vi "saveVI.vi"(8 "error in (no error)":errorcluster, 11 "PolymorphicInstance in":refnum<class "PolymorphicInstance.lvclass">) -> (0 "error out":errorcluster, 3 "PolymorphicInstance out":refnum<class "PolymorphicInstance.lvclass">)   [LabVIEW 2013, in "PolymorphicInstance.lvclass"]
uses:
  PolymorphicInstance.lvclass
  PolymorphicInstance.lvclass/PolymorphicInstance.ctl
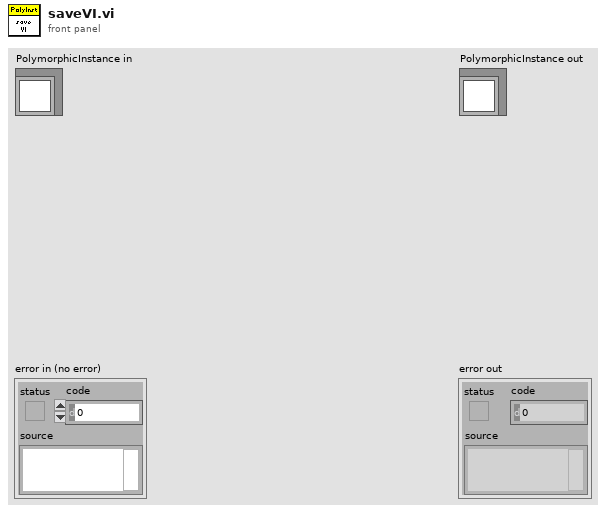
[diagram p1: front panel]
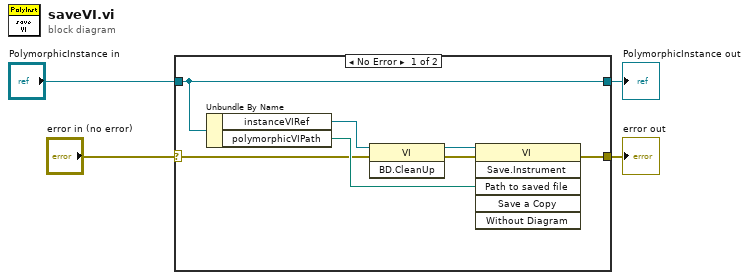
[diagram p0: block diagram]
diagram:
  n1 = case shown="No Error" "error in (no error)" {
    selector: "error in (no error)" -> [w6 w13]
    tunnel: [w5 w13] -> w3
    tunnel: [w11 w12] -> w1
    tunnel: "PolymorphicInstance in" -> [w11 w12]
    frame No Error {
      n2 = Unbundle By Name(w11) -> ("instanceVIRef"=w10:refnum<vi>, "polymorphicVIPath"=w8:path)
      n3 = invoke class="VI" method="BD.CleanUp"(reference=w10, error in=w6) -> (reference out=w9:refnum<vi>, error out=w7:errorcluster)  [unwired: 1 in, 1 out]
      n4 = invoke class="VI" method="Save.Instrument"(reference=w9, error in=w7, "Path to saved file"=w8) -> (error out=w5:errorcluster)  [unwired: 3 in, 5 out]
    }
    frame Error {
    }
  }
  "error out" <- w3
  "PolymorphicInstance out" <- w1
